vi "array - generate range.vi"(6 "N":i32=-1, 9 "df":dbl, 10 "freq max":dbl, 11 "freq min":dbl) -> (0 "Array":dbl[](array[numeric]), 2 "df out":dbl)   [LabVIEW 2018]
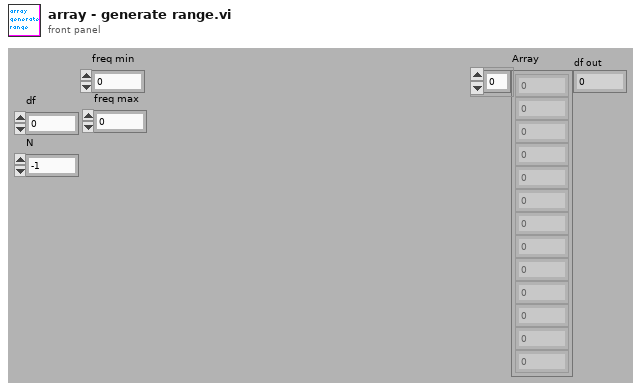
[diagram p1: front panel]
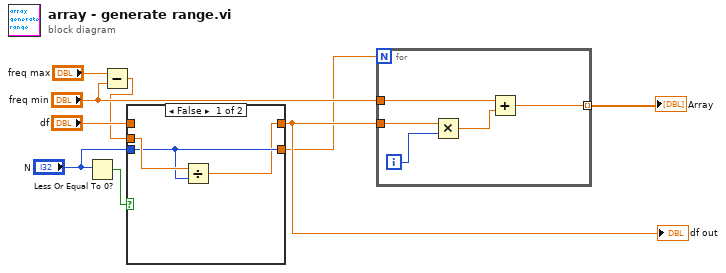
[diagram p0: block diagram]
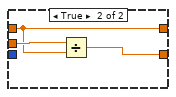
[diagram p2: hidden frame]
diagram:
  n1 = Less Or Equal To 0?(x="N") -> (x <= 0?=w6:bool)
  n2 = Subtract(x="freq max", y="freq min") -> (x-y=w3:dbl)
  n3 = case shown="False" w6 {
    tunnel: [w10 w14] -> w5
    tunnel: "df" -> [_ w14]
    tunnel: w3 -> [w12 w15]
    tunnel: [w11 w13] -> w2
    tunnel: "N" -> [w11 _]
    frame False {
      n4 = Divide(x=w12, y=w11) -> (x/y=w10:dbl)
    }
    frame True {
      n5 = Divide(x=w15, y=w14) -> (x/y=w13:dbl)
    }
  }
  "df out" <- w5
  n6 = for {
    N: w2 -> [_]
    tunnel: w5 -> [w19]
    tunnel: "freq min" -> [w17]
    tunnel: [w16] -> w7 mode=indexing
    i -> [w20]
    n7 = Multiply(x=w19, y=w20) -> (x*y=w18:dbl)
    n8 = Add(x=w17, y=w18) -> (x+y=w16:dbl)
  }
  "Array" <- w7
